vi "WaitForReceivedString.vi"(8 "error in (no error)":errorcluster, 10 "timeout in ms":i32=50, 11 "queue cluster":T1) -> (0 "error out":errorcluster, 1 "new value":bool, 2 "received string":string, 3 "queue cluster out":T1)   [LabVIEW 2014]
uses:
  typedefs/QueueCluster.ctl
  typedefs/clientStatus.ctl
panel:
  in  "keep semaphore":bool
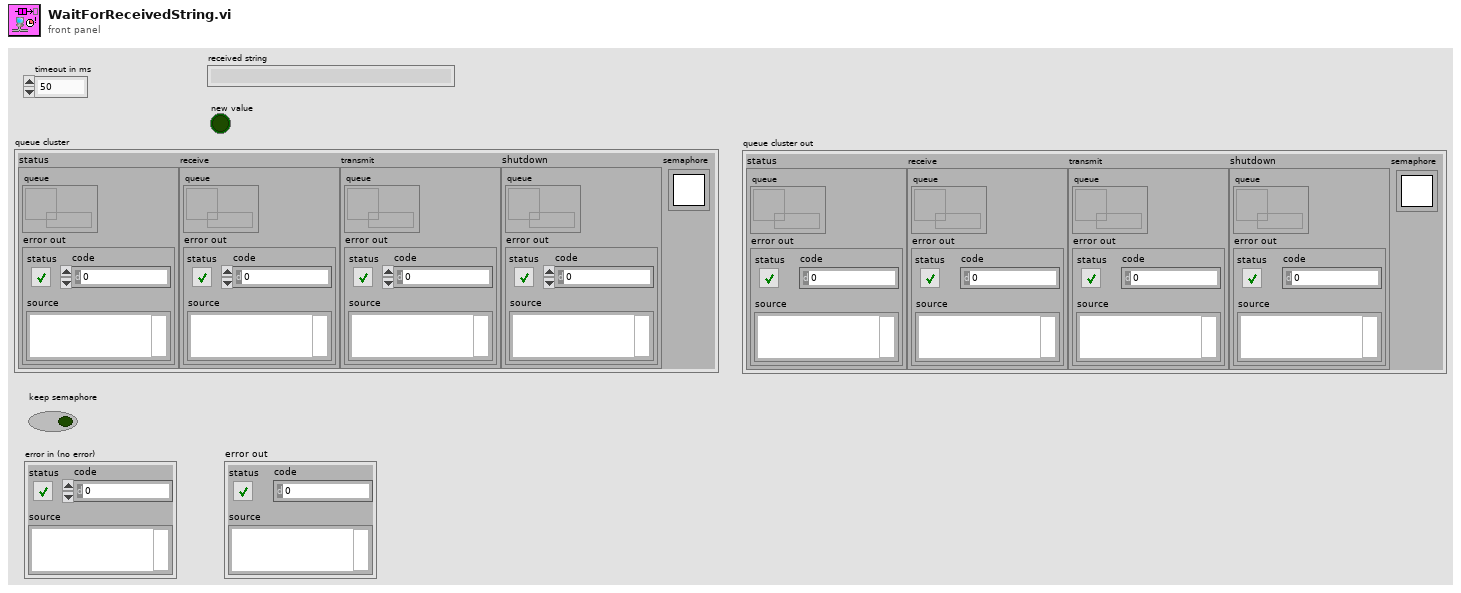
[diagram p1: front panel]
types:
  T1 = typedef "QueueCluster.ctl" = cluster{"status":cluster{"queue":refnum<queue>, "error out":errorcluster}, "receive":cluster{"queue":refnum<queue>, "error out":errorcluster}, "transmit":cluster{"queue":refnum<queue>, "error out":errorcluster}, "shutdown":cluster{"queue":refnum<queue>, "error out":errorcluster}, "semaphore":T2}
  T2 = typedef "Semaphore RefNum" = refnum<k1>
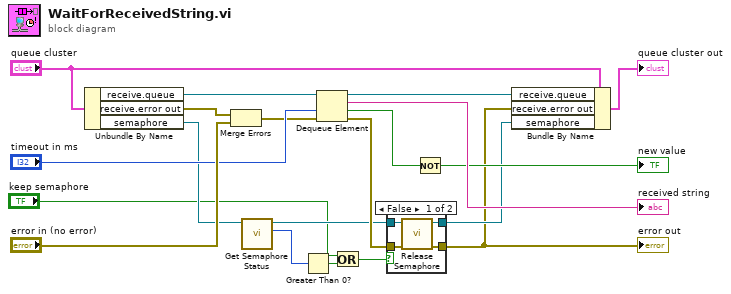
[diagram p0: block diagram]
diagram:
  n1 = Unbundle By Name("queue cluster") -> ("receive.queue"=w17:refnum<queue>, "receive.error out"=w16:errorcluster, "semaphore"=w5:T2)
  n2 = Merge Errors(w16, "error in (no error)") -> (w10:errorcluster)
  n3 = call <vilib>:"Get Semaphore Status.vi"("semaphore"=w5) -> ("# available"=w6:i32, "semaphore out"=w4:T2)  [unwired: 5 in, 4 out]
  n4 = Greater Than 0?(x=w6) -> (x > 0?=w3:bool)
  n5 = Dequeue Element(queue=w17, timeout in ms (-1)="timeout in ms", error in (no error)=w10) -> (queue out=w18:refnum<queue>, element=→"received string":string, timed out?=w11:bool, error out=w8:errorcluster)
  n6 = Or(x="keep semaphore", y=w3) -> (x .or. y?=w1:bool)
  n7 = case shown="False" w1 {
    tunnel: w4 -> [w24 w26]
    tunnel: [w23 w26] -> w9
    tunnel: w8 -> [w22 w25]
    tunnel: [w21 w25] -> w7
    frame False {
      n8 = call <vilib>:"Release Semaphore.vi"("error in (no error)"=w22, "semaphore"=w24) -> ("error out"=w21:errorcluster, "semaphore out"=w23:T2)  [unwired: 4 in]
    }
    frame True {
    }
  }
  "error out" <- w7
  n9 = Not(x=w11) -> (.not. x?=→"new value":bool)
  n10 = Bundle By Name(cluster="queue cluster", "receive.queue"=w18, "receive.error out"=w7, "semaphore"=w9) -> (→"queue cluster out":T1)
